vi "EncoderWithLimit.vi"(0 "Encoder B Channel":T2=enum."DIO 1", 1 "Encoder A Channel":T2, 2 "Reset Encoder?":bool, 5 "Invert Direction":bool, 7 "Decoding Type":T1=enum."4x", 9 "DistancePerCount (deg)":dbl=0.288, 11 "Minimum Rate":dbl=20.0, 12 "Number Samples to Average":u8=1 min=1 max=128, 13 "Wheel diameter (in)":dbl=6.0) -> (3 "Encoder Direction":string, 4 "Encoder Rate (deg/sec)":dbl, 6 "Encoder Alarm Status":string, 8 "dReached":bool, 10 "Distance (in)":dbl, 14 "Current angle (deg)":dbl(knob) scale=0.0..360.0, 15 "Revolutions":dbl)   [LabVIEW 2019]
uses:
  <vilib>/Rock Robotics/SystemInterfaces/DIO/FPGA_DIOChannel.ctl
  <vilib>/Rock Robotics/WPI/Encoder/WPI_EncoderType.ctl
  <vilib>/Rock Robotics/WPI/Counter/WPI_CounterDigitalInputToDigitalSource.vi
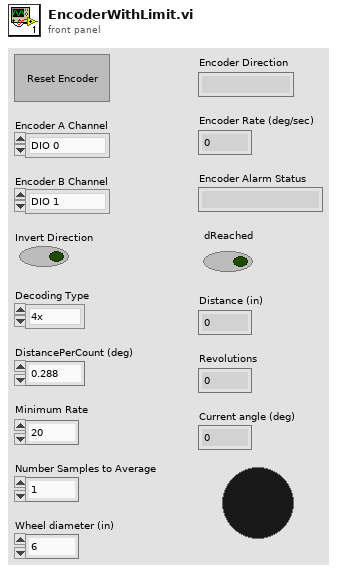
[diagram p1: front panel]
types:
  T1 = typedef "WPI_EncoderType.ctl" = enum16{"1x", "2x", "4x"}
  T2 = typedef "FPGA_DIOChannel.ctl" = enum8{"DIO 0", "DIO 1", "DIO 2", "DIO 3", "DIO 4", "DIO 5", "DIO 6", "DIO 7", "DIO 8", "DIO 9", "DIO MXP 0", "DIO MXP 1", "DIO MXP 2", "DIO MXP 3", "DIO MXP 4", "DIO MXP 5", "DIO MXP 6", "DIO MXP 7", "DIO MXP 8", "DIO MXP 9", "DIO MXP 10", "DIO MXP 11", "DIO MXP 12", "DIO MXP 13", "DIO MXP 14", "DIO MXP 15", "SPI Port CS1", "SPI Port CS2", "SPI Port CS3", "SPI Port MISO", "SPI Port MOSI", "Invalid"}
  T3 = typedef "WPI_DigitalInputDevRef.ctl" = cluster{"DevStatus":errorcluster, "DIO Channel":T2}
  T4 = typedef "FPGA_CounterEncoderSourceConvertionLVSourceType.ctl" = cluster{"DevStatus":errorcluster, "AnalogTriggerMode?":bool, "DigitalMode":cluster{"DIO Channel":T5}, "AnalogTriggerMode":cluster{"AnalogTriggerIndex":T6, "OutputType":T7}}
  T5 = typedef "FPGA_DIODigitalSourceChannel.ctl" = enum8{"DIO 0", "DIO 1", "DIO 2", "DIO 3", "DIO 4", "DIO 5", "DIO 6", "DIO 7", "DIO 8", "DIO 9", "DIO MXP 0", "DIO MXP 1", "DIO MXP 2", "DIO MXP 3", "DIO MXP 4", "DIO MXP 5", "DIO MXP 6", "DIO MXP 7", "DIO MXP 8", "DIO MXP 9", "DIO MXP 10", "DIO MXP 11", "DIO MXP 12", "DIO MXP 13", "DIO MXP 14", "DIO MXP 15", "SPI Port CS1", "SPI Port CS2", "SPI Port CS3", "SPI Port MISO", "SPI Port MOSI", "Disabled"}
  T6 = typedef "FPGA_AnalogTriggerIndex.ctl" = enum8{"Trig 0", "Trig 1", "Trig 2", "Trig 3", "Trig 4", "Trig 5", "Trig 6", "Trig 7", "Invalid"}
  T7 = typedef "FPGA_AnalogTriggerOutType.ctl" = enum16{"InWindow", "TriggerState", "Rising", "Falling"}
  T8 = typedef "WPI_EncoderDevRef.ctl" = cluster{"DevStatus":errorcluster, "EncoderIndex":T9, "CounterIndex":T10, "DistancePerCount":dbl, "Decoding Type":T1}
  T9 = typedef "FPGA_EncoderIdx.ctl" = enum8{"Enc 0", "Enc 1", "Enc 2", "Enc 3", "Enc 4", "Enc 5", "Enc 6", "Enc 7", "Invalid"}
  T10 = typedef "FPGA_CounterCtrSystemIndex.ctl" = enum8{"Ctr 0", "Ctr 1", "Ctr 2", "Ctr 3", "Ctr 4", "Ctr 5", "Ctr 6", "Ctr 7", "Invalid"}
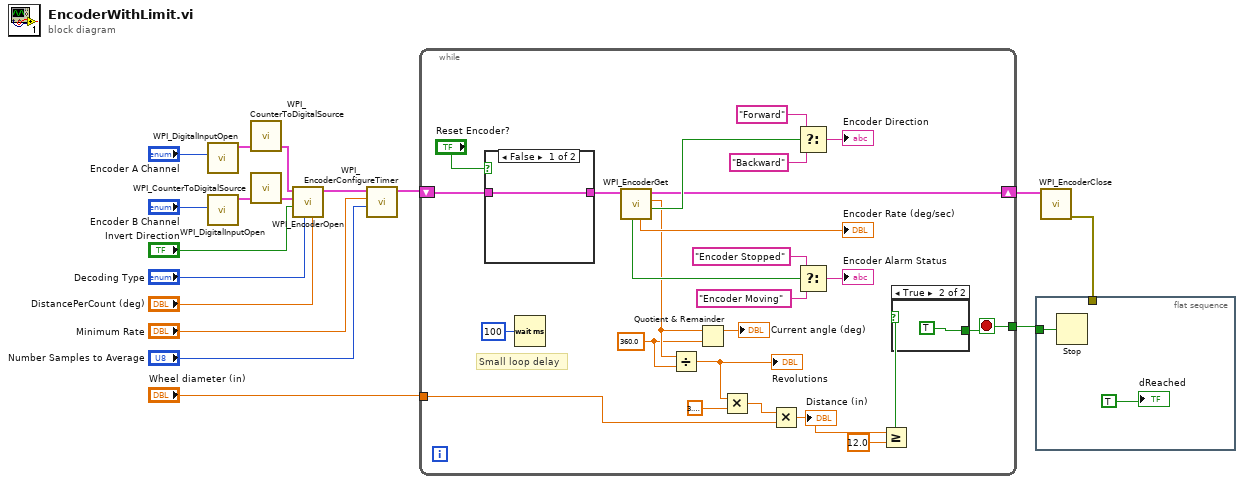
[diagram p0: block diagram]
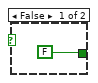
[diagram p2: hidden frame]
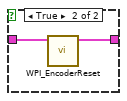
[diagram p3: hidden frame]
diagram:
  n1 = call <vilib>:"WPI_DigitalInputOpen.vi"("DIO Channel"="Encoder A Channel") -> ("DigitalInputDevRef"=w14:T3)  [unwired: 1 in, 9 out]
  n2 = call <vilib>:"WPI_DigitalInputOpen.vi"("DIO Channel"="Encoder B Channel") -> ("DigitalInputDevRef"=w15:T3)  [unwired: 1 in, 9 out]
  n3 = call-poly <vilib>:"WPI_CounterToDigitalSource.vi"("DigitalInputDevRef"=w14) -> ("Digital Source"=w13:T4)  [unwired: 6 out]
  n4 = call-poly <vilib>:"WPI_CounterToDigitalSource.vi"("DigitalInputDevRef"=w15) -> ("Digital Source"=w16:T4)  [unwired: 6 out]
  n5 = call <vilib>:"WPI_EncoderOpen.vi"("DistancePerCount"="DistancePerCount (deg)", "Decoding Type"="Decoding Type", "Invert Direction (False)"="Invert Direction", "BSource"=w16, "ASource"=w13) -> ("EncoderDevRef"=w6:T8)  [unwired: 3 in, 3 out]
  n6 = call <vilib>:"WPI_EncoderConfigureTimer.vi"("Number Samples to Average"="Number Samples to Average", "Minimum Rate"="Minimum Rate", "EncoderDevRef"=w6) -> ("EncoderDevRef"=w7:T8)  [unwired: 1 in, 7 out]
  n7 = while {
    shift-right: [w35] -> w17
    shift-left: w7 -> [w40]
    tunnel: "Wheel diameter (in)" -> [w25]
    tunnel: [w21] -> w1
    stop <- w21 stop-if-true
    w27 = 360.0 ("y")
    # "Small loop delay"
    n8 = case shown="False" "Reset Encoder?" {
      tunnel: w40 -> [w45 w47]
      tunnel: [w45 w46] -> w38
      frame False {
      }
      frame True {
        n9 = call <vilib>:"WPI_EncoderReset.vi"("EncoderDevRef"=w47) -> ("EncoderDevRef"=w46:T8)  [unwired: 1 in, 9 out]
      }
    }
    n10 = Wait (ms)(milliseconds to wait=u32 100) -> ()  [unwired: 1 out]
    n11 = call <vilib>:"WPI_EncoderGet.vi"("EncoderDevRef"=w38) -> ("Direction"=w37:bool, "Distance"=w28:dbl, "EncoderDevRef"=w35:T8, "Rate"=→"Encoder Rate (deg/sec)":dbl, "Stopped"=w36:bool)  [unwired: 1 in, 5 out]
    n12 = Divide(x=w28, y=w27) -> (x/y=w22:dbl)
    "Revolutions" <- w22
    n13 = Quotient & Remainder(x=w28, y=w27) -> (x-y*floor(x/y)=→"Current angle (deg)":dbl)  [unwired: 1 out]
    n14 = Multiply(x=w22, y=3.141592653589793) -> (x*y=w24:dbl)
    n15 = Multiply(x=w24, y=w25) -> (x*y=w20:dbl)
    "Distance (in)" <- w20
    n16 = Select(t="Forward", s=w37, f="Backward") -> (s? t:f=→"Encoder Direction":string)
    n17 = Select(t="Encoder Stopped", s=w36, f="Encoder Moving") -> (s? t:f=→"Encoder Alarm Status":string)
    n18 = Greater Or Equal?(x=w20, y=12.0) -> (x >= y?=w18:bool)
    n19 = case shown="True" w18 {
      tunnel: [FALSE TRUE] -> w21
      frame False {
      }
      frame True {
      }
    }
  }
  n20 = flat-sequence {
    tunnel: w1 -> [w49]
    tunnel: w2 -> [_]
    frame #0 {
      n21 = Stop(stop? (T)=w49) -> ()
      "dReached" <- TRUE
    }
  }
  n22 = call <vilib>:"WPI_EncoderClose.vi"("EncoderDevRef"=w17) -> ("error out"=w2:errorcluster)  [unwired: 2 in, 8 out]
